vi "ReadSizeNchwMat.vi"   [LabVIEW 2020, in "OpenLvVision_OpenCv.lvlib"]
uses:
  OpenLvVision_OpenCv.lvlib
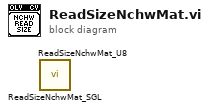
[diagram p0: block diagram]
diagram:
  n1 = call "ReadSizeNchwMat_SGL.vi"() -> ()  [unwired: 6 in, 6 out]
  n2 = call "ReadSizeNchwMat_U8.vi"() -> ()  [unwired: 6 in, 6 out]
